vi "WLAN - TV - OPPO - RW - UTIL - TestVectors_11A.vi"(0 "IQComp_11AG OFDM":T1={"Standard"=0, "OFDM Advanced Controls"={"OFDM Auto Compute Acquisition Length Enabled"=0, "OFDM Maximum Symbols Used"=0, "OFDM Time Tracking Enabled"=0, "OFDM Channel Tracking Enabled"=0, "OFDM Amplitude Tracking Enabled"=1, "OFDM CFO Estimation Method"=0, "OFDM Phase Tracking Method"=0, "OFDM Header Detection Enabled"=0, "OFDM MAC FCS Check Enabled"=0, "#Avg"=0, "#Iterations"=10}, "Measurement  Enabled ?"=FALSE, "#Packets"=0, "Center Frequency(Hz)"=0.0, "Power Level(dBm)"=0.0, "Payload Control"={"OFDM Data Rate (Mbps)"=0, "OFDM Payload Length (bytes)"=0, "Idle Interval (s)"=0.0}} {"Payload Control"."OFDM Data Rate (Mbps)" items=["6", "9", "12", "18", "24", "36", "48", "54"]; "Center Frequency(Hz)" format="%#_6p"; "OFDM Advanced Controls"."OFDM Phase Tracking Method" items=["Standard", "Instantaneous", "None", "Standard with Cubic Spline Fit"]; "OFDM Advanced Controls"."OFDM CFO Estimation Method" items=["Preamble Only", "Preamble and Data"]; "OFDM Advanced Controls"."OFDM Channel Tracking Enabled" items=["False", "True"]; "OFDM Advanced Controls"."OFDM Amplitude Tracking Enabled" items=["False", "True"]; "OFDM Advanced Controls"."OFDM Time Tracking Enabled" items=["True"=1, "False"=0]; "OFDM Advanced Controls"."OFDM Auto Compute Acquisition Length Enabled" items=["False", "True"]; "OFDM Advanced Controls"."OFDM MAC FCS Check Enabled" items=["False", "True"]; "OFDM Advanced Controls"."OFDM Header Detection Enabled" items=["False", "True"]; "Standard" items=["80211A/G/J/P OFDM", "80211B/G DSSS", "80211G DSSSOFDM", "80211N MIMOOFDM", "80211AC MIMOOFDM"]}, 9 "TV Paramaters":T3) -> (6 "TV":string[][](array[string]), 8 "Measure Config":string[][](array[string]))   [LabVIEW 2012]
uses:
  Includes/WLAN - TV - RW - INC - TV_Parameters.ctl
  Includes/WLAN - TV - OPPO - RW - INC - TV_IQComposite_11A.ctl
  Includes/WLAN - TV - RW - INC - TV_OFDM Demod.ctl
  Includes/WLAN - TV - RW - INC - Tx_Meas_Settings_OFDM_String.ctl
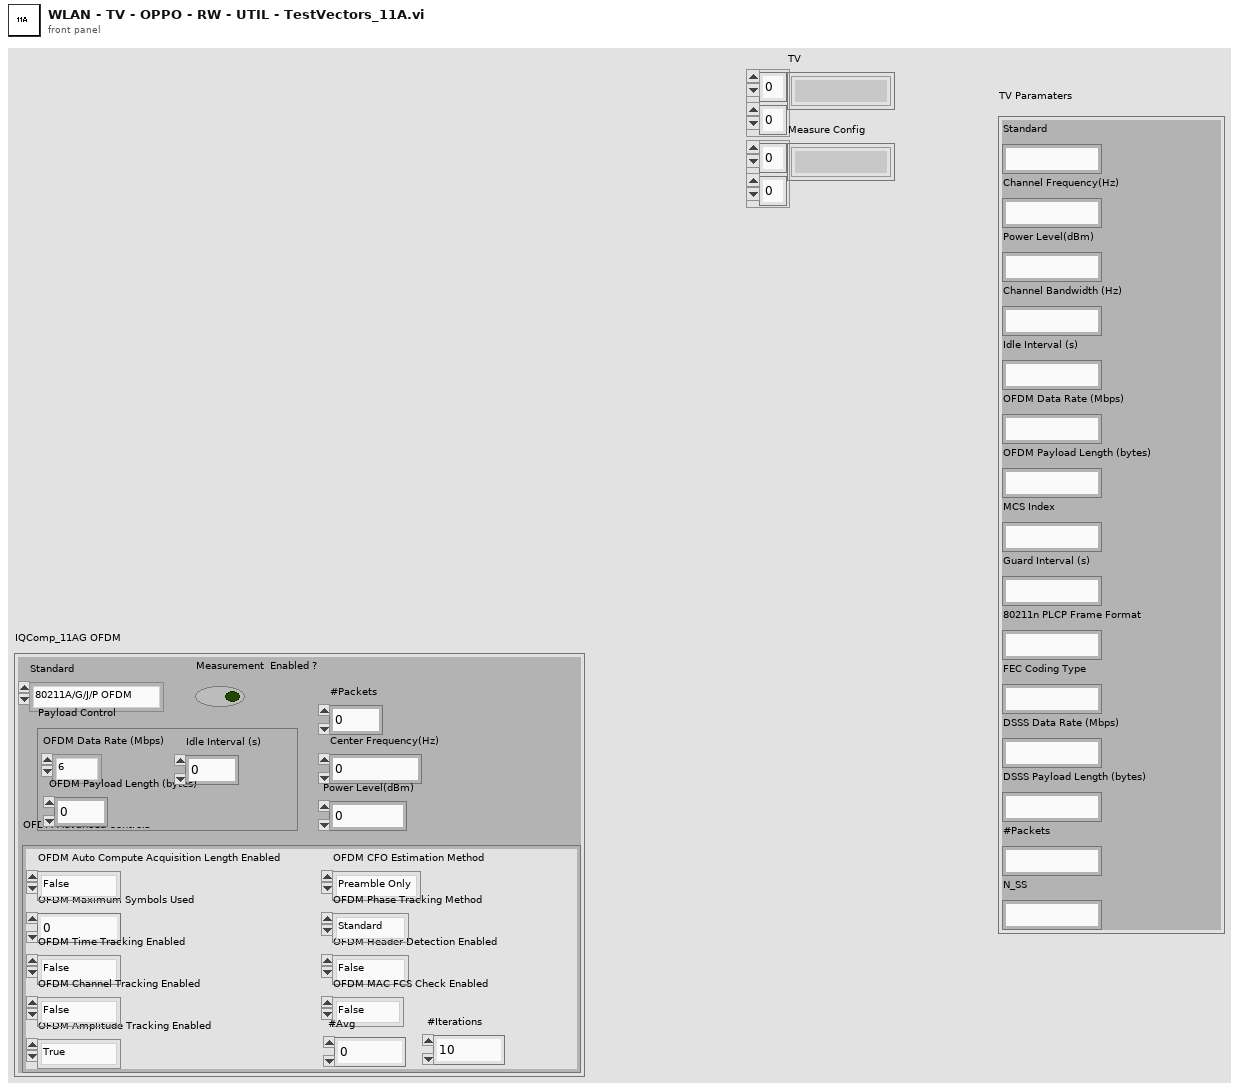
[diagram p1: front panel]
types:
  T1 = typedef "WLAN - TV - OPPO - RW - INC - TV_IQComposite_11A.ctl" = cluster{"Standard":i32, "OFDM Advanced Controls":T2, "Measurement  Enabled ?":bool, "#Packets":i32, "Center Frequency(Hz)":dbl, "Power Level(dBm)":dbl, "Payload Control":cluster{"OFDM Data Rate (Mbps)":i32, "OFDM Payload Length (bytes)":i32, "Idle Interval (s)":dbl}}
  T2 = typedef "WLAN - TV - RW - INC - TV_OFDM Demod.ctl" = cluster{"OFDM Auto Compute Acquisition Length Enabled":i32, "OFDM Maximum Symbols Used":i32, "OFDM Time Tracking Enabled":i32, "OFDM Channel Tracking Enabled":i32, "OFDM Amplitude Tracking Enabled":i32, "OFDM CFO Estimation Method":i32, "OFDM Phase Tracking Method":i32, "OFDM Header Detection Enabled":i32, "OFDM MAC FCS Check Enabled":i32, "#Avg":i32, "#Iterations":i32}
  T3 = typedef "WLAN - TV - RW - INC - TV_Parameters.ctl" = cluster{"Standard ":string, "Channel Frequency(Hz)":string, "Power Level(dBm)":string, "Channel Bandwidth (Hz)":string, "Idle Interval (s)":string, "OFDM Data Rate (Mbps)":string, "OFDM Payload Length (bytes)":string, "MCS Index":string, "Guard Interval (s)":string, "80211n PLCP Frame Format":string, "FEC Coding Type":string, "DSSS Data Rate (Mbps)":string, "DSSS Payload Length (bytes)":string, "#Packets":string, "N_SS":string}
  T4 = typedef "WLAN - TV - RW - INC - Tx_Meas_Settings_OFDM_String.ctl" = cluster{"OFDM Auto Compute Acquisition Length Enabled":string, "OFDM Maximum Symbols Used":string, "OFDM Time Tracking Enabled":string, "OFDM Channel Tracking Enabled":string, "OFDM Amplitude Tracking Enabled":string, "OFDM CFO Estimation Method":string, "OFDM Phase Tracking Method":string, "OFDM Header Detection Enabled":string, "OFDM MAC FCS Check Enabled":string, "#Avg":string, "#Iterations":string}
  T5 = cluster{"OFDM Data Rate (Mbps)":i32, "OFDM Payload Length (bytes)":i32, "Idle Interval (s)":dbl}
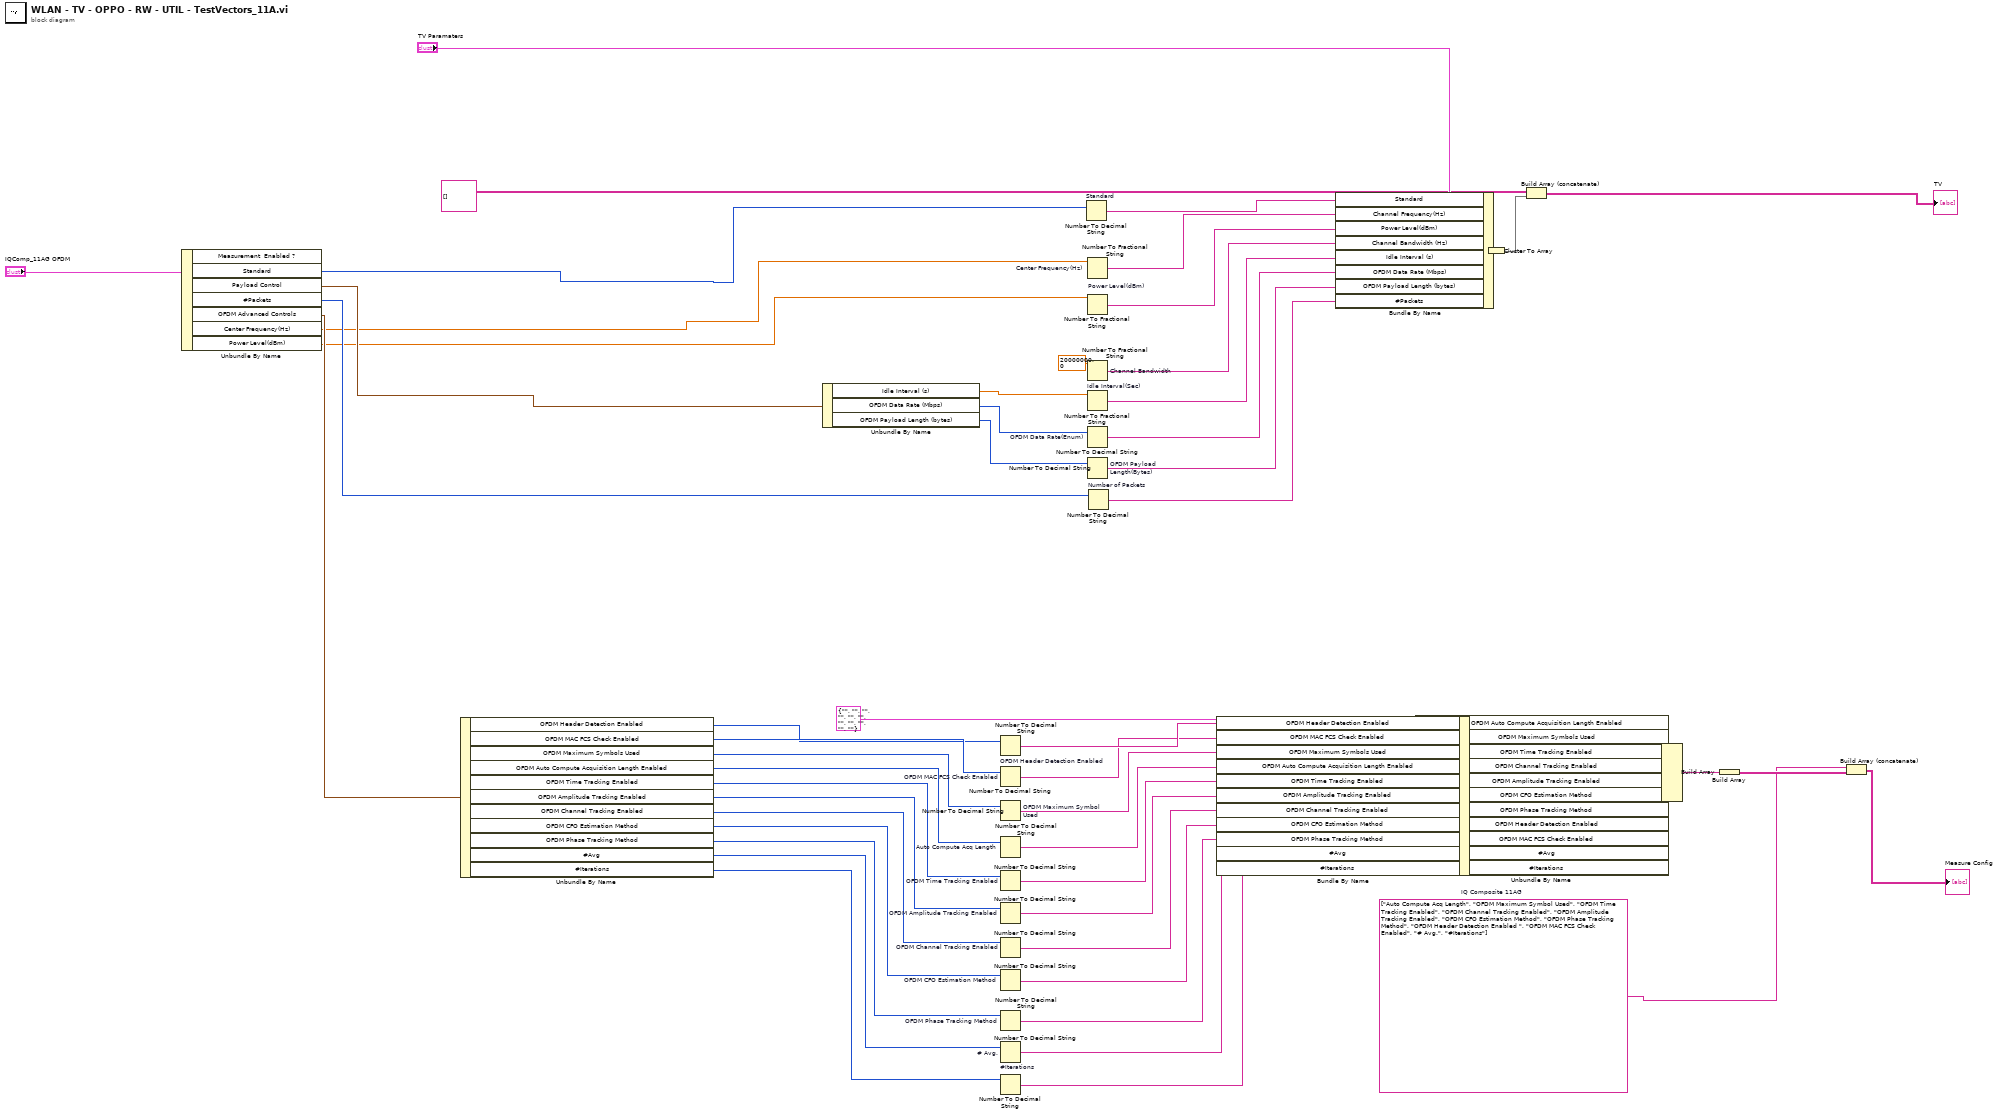
[diagram p0: block diagram]
diagram:
  w19 = string[] ["Auto Compute Acq Length", "OFDM Maximum Symbol Used", "OFDM Time Tracking Enabled", "OFDM Channel Tracking Enabled", "OFDM Amplitude Tracking Enabled", "OFDM CFO Estimation Method", "OFDM Phase Tracking Method", "OFDM Header Detection Enabled ", "OFDM MAC FCS Check Enabled", "# Avg.", "#Iterations"]  # IQ Composite 11AG
  n1 = Unbundle By Name("IQComp_11AG OFDM") -> ("Standard"=w63:i32, "Payload Control"=w60:T5, "#Packets"=w58:i32, "OFDM Advanced Controls"=w59:T2, "Center Frequency(Hz)"=w16:dbl, "Power Level(dBm)"=w15:dbl)  [unwired: 1 out]
  n2 = Unbundle By Name(w59) -> ("OFDM Header Detection Enabled"=w47:i32, "OFDM MAC FCS Check Enabled"=w48:i32, "OFDM Maximum Symbols Used"=w49:i32, "OFDM Auto Compute Acquisition Length Enabled"=w50:i32, "OFDM Time Tracking Enabled"=w51:i32, "OFDM Amplitude Tracking Enabled"=w52:i32, "OFDM Channel Tracking Enabled"=w53:i32, "OFDM CFO Estimation Method"=w54:i32, "OFDM Phase Tracking Method"=w55:i32, "#Avg"=w56:i32, "#Iterations"=w57:i32)
  n3 = Unbundle By Name(w60) -> ("Idle Interval (s)"=w4:dbl, "OFDM Data Rate (Mbps)"=w6:i32, "OFDM Payload Length (bytes)"=w5:i32)
  n4 = Number To Decimal String "OFDM Header Detection Enabled"(number=w47) -> (decimal integer string=w45:string)  [unwired: 1 in]
  n5 = Number To Decimal String "OFDM MAC FCS Check Enabled"(number=w48) -> (decimal integer string=w44:string)  [unwired: 1 in]
  n6 = Number To Decimal String "OFDM Maximum Symbol Used"(number=w49) -> (decimal integer string=w43:string)  [unwired: 1 in]
  n7 = Number To Decimal String "Auto Compute Acq Length"(number=w50) -> (decimal integer string=w42:string)  [unwired: 1 in]
  n8 = Number To Decimal String "OFDM Time Tracking Enabled"(number=w51) -> (decimal integer string=w41:string)  [unwired: 1 in]
  n9 = Number To Decimal String "OFDM Amplitude Tracking Enabled"(number=w52) -> (decimal integer string=w40:string)  [unwired: 1 in]
  n10 = Number To Decimal String "OFDM Channel Tracking Enabled"(number=w53) -> (decimal integer string=w35:string)  [unwired: 1 in]
  n11 = Number To Decimal String "OFDM CFO Estimation Method"(number=w54) -> (decimal integer string=w36:string)  [unwired: 1 in]
  n12 = Number To Decimal String "OFDM Phase Tracking Method"(number=w55) -> (decimal integer string=w37:string)  [unwired: 1 in]
  n13 = Number To Decimal String "# Avg."(number=w56) -> (decimal integer string=w38:string)  [unwired: 1 in]
  n14 = Number To Decimal String "#Iterations"(number=w57) -> (decimal integer string=w39:string)  [unwired: 1 in]
  n15 = Number To Decimal String "Standard"(number=w63) -> (decimal integer string=w7:string)  [unwired: 1 in]
  n16 = Number To Fractional String "Center Frequency(Hz)"(number=w16) -> (F-format string=w8:string)  [unwired: 3 in]
  n17 = Number To Fractional String "Power Level(dBm)"(number=w15) -> (F-format string=w9:string)  [unwired: 3 in]
  n18 = Number To Fractional String "Channel Bandwidth"(number=20000000.0) -> (F-format string=w10:string)  [unwired: 3 in]
  n19 = Number To Fractional String "Idle Interval(Sec)"(number=w4) -> (F-format string=w11:string)  [unwired: 3 in]
  n20 = Number To Decimal String "OFDM Data Rate(Enum)"(number=w6) -> (decimal integer string=w12:string)  [unwired: 1 in]
  n21 = Number To Decimal String "OFDM Payload Length(Bytes)"(number=w5) -> (decimal integer string=w13:string)  [unwired: 1 in]
  n22 = Number To Decimal String "Number of Packets"(number=w58) -> (decimal integer string=w3:string)  [unwired: 1 in]
  n23 = Bundle By Name(cluster=T4 {"OFDM Auto Compute Acquisition Length Enabled"="", "OFDM Maximum Symbols Used"="", "OFDM Time Tracking Enabled"="", "OFDM Channel Tracking Enabled"="", "OFDM Amplitude Tracking Enabled"="", "OFDM CFO Estimation Method"="", "OFDM Phase Tracking Method"="", "OFDM Header Detection Enabled"="", "OFDM MAC FCS Check Enabled"="", "#Avg"="", "#Iterations"=""} ("OFDM Measurement Settings"), "OFDM Header Detection Enabled"=w45, "OFDM MAC FCS Check Enabled"=w44, "OFDM Maximum Symbols Used"=w43, "OFDM Auto Compute Acquisition Length Enabled"=w42, "OFDM Time Tracking Enabled"=w41, "OFDM Amplitude Tracking Enabled"=w40, "OFDM Channel Tracking Enabled"=w35, "OFDM CFO Estimation Method"=w36, "OFDM Phase Tracking Method"=w37, "#Avg"=w38, "#Iterations"=w39) -> (w34:T4)
  n24 = Bundle By Name(cluster="TV Paramaters", "Standard"=w7, "Channel Frequency(Hz)"=w8, "Power Level(dBm)"=w9, "Channel Bandwidth (Hz)"=w10, "Idle Interval (s)"=w11, "OFDM Data Rate (Mbps)"=w12, "OFDM Payload Length (bytes)"=w13, "#Packets"=w3) -> (w2:T3)
  n25 = Unbundle By Name(w34) -> ("OFDM Auto Compute Acquisition Length Enabled"=w33:string, "OFDM Maximum Symbols Used"=w32:string, "OFDM Time Tracking Enabled"=w31:string, "OFDM Channel Tracking Enabled"=w30:string, "OFDM Amplitude Tracking Enabled"=w29:string, "OFDM CFO Estimation Method"=w28:string, "OFDM Phase Tracking Method"=w27:string, "OFDM Header Detection Enabled"=w26:string, "OFDM MAC FCS Check Enabled"=w25:string, "#Avg"=w24:string, "#Iterations"=w23:string)
  n26 = Cluster To Array(cluster=w2) -> (array=w1:string[])
  n27 = Build Array (concatenate)(string[][] [] ("appended array"), w1) -> (→"TV":string[][])
  n28 = Build Array(w33, w32, w31, w30, w29, w28, w27, w26, w25, w24, w23) -> (w22:string[])
  n29 = Build Array(w22) -> (w20:string[][])
  n30 = Build Array (concatenate)(w19, w20) -> (→"Measure Config":string[][])
